vi "Read PID Loops.vi"(8 "error in (no error)":errorcluster, 11 "Tagbus PID Module configuration in":refnum<class "PID Module configuration.lvclass">) -> (0 "error out":errorcluster, 2 "PID Loops":refnum<class "PID Loop.lvclass">[](array[class]), 3 "Tagbus PID Module configuration out":refnum<class "PID Module configuration.lvclass">)   [LabVIEW 2013, in "PID Module configuration.lvclass"]
doc: "This VI returns the array of PID Loops associated with the Module Configuration."
uses:
  PID Module configuration.lvclass
  PID Loop.lvclass
  PID Module configuration.lvclass/PID Module configuration.ctl
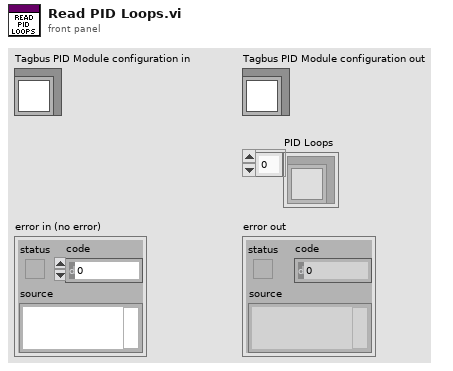
[diagram p1: front panel]
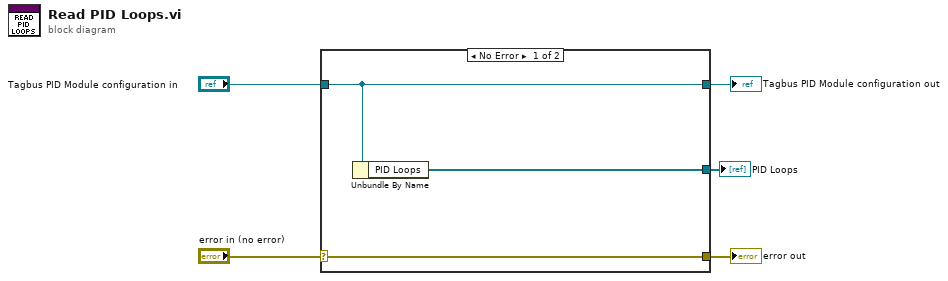
[diagram p0: block diagram]
diagram:
  n1 = case shown="No Error" "error in (no error)" {
    selector: "error in (no error)" -> [w8 w9]
    tunnel: [w8 w9] -> w4
    tunnel: [w7 w10] -> w2
    tunnel: "Tagbus PID Module configuration in" -> [w7 w10]
    tunnel: [w6 _] -> w1
    frame No Error {
      n2 = Unbundle By Name(w7) -> ("PID Loops"=w6:refnum<class "PID Loop.lvclass">[])
    }
    frame Error {
    }
  }
  "error out" <- w4
  "Tagbus PID Module configuration out" <- w2
  "PID Loops" <- w1
